vi "zs_goal.vi"(8 "Yaw (z)":dbl, 10 "Point.y":dbl, 11 "Point.x":dbl) -> (3 "msg out":string)   [LabVIEW 2014]
uses:
  ctl/pose.ctl
  ctl/orientation.ctl
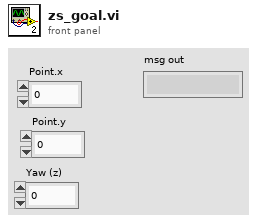
[diagram p1: front panel]
types:
  T1 = typedef "orientation.ctl" = cluster{"Roll (y)":dbl, "Pitch (x)":dbl, "Yaw (z)":dbl}
  T2 = typedef "pose.ctl" = cluster{"Point":cluster{"x":dbl, "y":dbl, "z":dbl}, "Quaternion":cluster{"x":dbl, "y":dbl, "z":dbl, "w":dbl}}
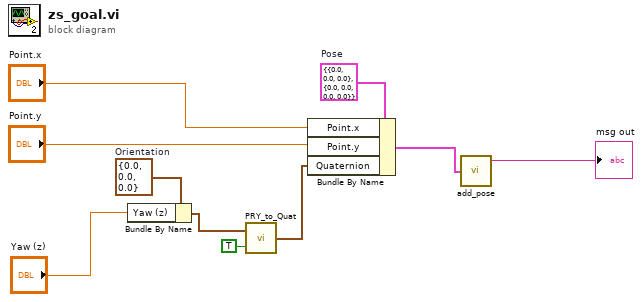
[diagram p0: block diagram]
diagram:
  w5 = T1 {"Roll (y)"=0.0, "Pitch (x)"=0.0, "Yaw (z)"=0.0}  # Orientation
  w8 = T2 {"Point"={"x"=0.0, "y"=0.0, "z"=0.0}, "Quaternion"={"x"=0.0, "y"=0.0, "z"=0.0, "w"=0.0}}  # Pose
  n1 = Bundle By Name(cluster=w5, "Yaw (z)"="Yaw (z)") -> (w7:T1)
  n2 = call <vilib>:"PRY_to_Quat.vi"("From Degrees? (T)"=TRUE, "Orientation"=w7) -> ("Quaternion"=w3:cluster{"x":dbl, "y":dbl, "z":dbl, "w":dbl})
  n3 = Bundle By Name(cluster=w8, "Point.x"="Point.x", "Point.y"="Point.y", "Quaternion"=w3) -> (w2:T2)
  n4 = call <vilib>:"add_pose.vi"("Pose"=w2) -> ("msg out"=→"msg out":string)  [unwired: 4 in]
